vi "datetimestring for folder name.vi"() -> (0 "concatenated string":string)   [LabVIEW 2024]
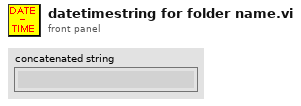
[diagram p1: front panel]
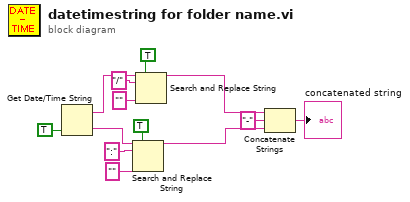
[diagram p0: block diagram]
diagram:
  n1 = Get Date/Time String(want seconds? (F)=TRUE) -> (date string=w6:string, time string=w5:string)  [unwired: 2 in]
  n2 = Search and Replace String(replace all?=TRUE ("replace all? (F)"), input string=w5, search string=":", replace string="" ("replace string (\"\")")) -> (result string=w3:string)  [unwired: 4 in, 3 out]
  n3 = Search and Replace String(replace all?=TRUE ("replace all? (F)"), input string=w6, search string="/", replace string="" ("replace string (\"\")")) -> (result string=w4:string)  [unwired: 4 in, 3 out]
  n4 = Concatenate Strings(w4, "-" ("string"), w3) -> (→"concatenated string":string)
